vi "FPGA Main.vi"() -> ()   [LabVIEW 2026]
uses:
  <vilib>/rvi/DataTransferAndStorage/Container/XNode/niFpgaContainer.xnode
  <vilib>/eio/EIONode/EIONode.xnode
  <vilib>/rvi/eio/common/nirviEmuTemplateMethod_errors.vi
  <vilib>/rvi/interface/RandomDataEmulation/nirviRandomDataFpgaReadWriteTemplate.vi
panel:
  in  "loop time [us]":u32=20
  out "from RT underflow?":bool
  out "to RT overflow?":bool
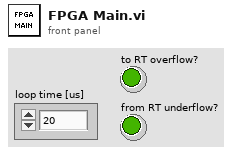
[diagram p1: front panel]
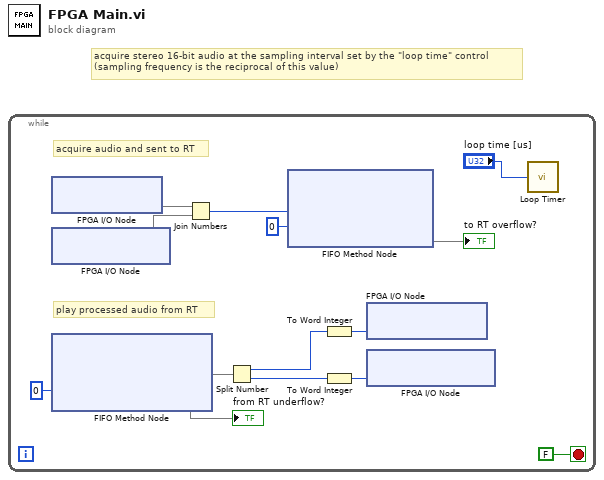
[diagram p0: block diagram]
diagram:
  # "acquire stereo 16-bit audio at the sampling interval set by the \"loop time\" control\n(sampling frequency is the reciprocal of this value)"
  n1 = while {
    stop <- FALSE stop-if-true
    # "play processed audio from RT"
    # "acquire audio and sent to RT"
    n2 = xnode "FPGA I/O Node"() -> ("AudioIn/Left"=w10)  [unwired: 1 in, 1 out]
    n3 = xnode "FPGA I/O Node"() -> ("AudioIn/Right"=w9)  [unwired: 1 in, 1 out]
    n4 = xnode ("FIFO Method Node")("Timeout"=0) -> ("Element"=w7, "Timed Out?"=→"from RT underflow?")  [unwired: 1 in, 1 out]
    n5 = Join Numbers(hi=w10, lo=w9) -> ((hi.lo)=w8:u32)
    n6 = Split Number(x=w7) -> (hi(x)=w4:u16, lo(x)=w3:u16)
    n7 = xnode "FIFO Method Node"("Element"=w8, "Timeout"=0) -> ("Timed Out?"=→"to RT overflow?")  [unwired: 1 in, 1 out]
    n8 = To Word Integer(number=w4) -> (16bit integer=w6:i16)
    n9 = To Word Integer(number=w3) -> (16bit integer=w5:i16)
    n10 = xnode "FPGA I/O Node"("AudioOut/Left"=w6) -> ()  [unwired: 1 in, 1 out]
    n11 = xnode "FPGA I/O Node"("AudioOut/Right"=w5) -> ()  [unwired: 1 in, 1 out]
    n12 = call "Loop Timer"("Count(uSec)"="loop time [us]") -> ()  [unwired: 1 out]
  }
